vi "Configure Device.vi"(8 "error in (no error)":errorcluster, 10 "Max beams":dbl, 11 "Device in":refnum<class "PIC-Device.lvclass">) -> (0 "error out":errorcluster, 3 "Device out":refnum<class "PIC-Device.lvclass">)   [LabVIEW 2020, in "PIC-Device.lvclass"]
doc: "Interface for configuring the device for testing"
uses:
  PIC-Device.lvclass
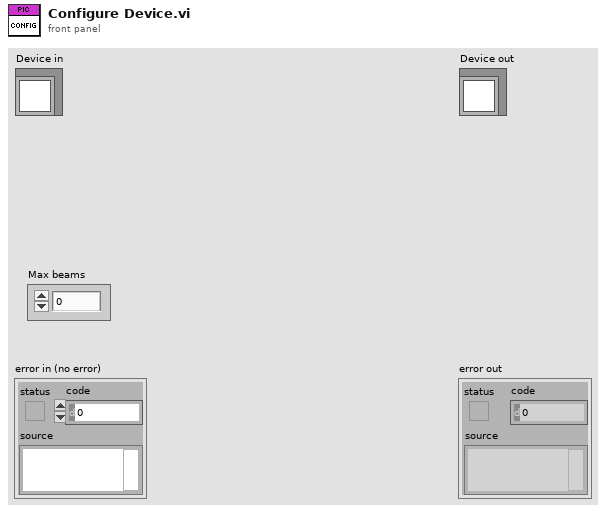
[diagram p1: front panel]
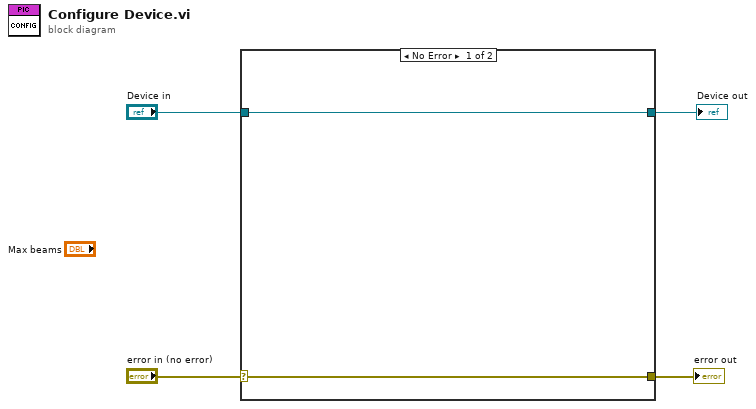
[diagram p0: block diagram]
diagram:
  n1 = case shown="No Error" "error in (no error)" {
    selector: "error in (no error)" -> [w5 w8]
    tunnel: [w5 w8] -> w3
    tunnel: [w6 w7] -> w1
    tunnel: "Device in" -> [w6 w7]
    frame No Error {
    }
    frame Error {
    }
  }
  "error out" <- w3
  "Device out" <- w1
